vi "Log Error.vi"(8 "error in (no error)":errorcluster, 9 "error":errorcluster, 10 "state":T1, 11 "Dispatcher in":refnum<class "Dispatcher Thread.lvclass">) -> (0 "error out":errorcluster, 3 "Dispatcher out":refnum<class "Dispatcher Thread.lvclass">)   [LabVIEW 2017, in "DSF Core.lvlib" / "Dispatcher Thread.lvclass"]
uses:
  Dispatcher Thread.lvclass
  C:/Git/DSF/Core/Classes/Thread/Thread.lvclass
  Interface/Dispatcher/Command.ctl
  Thread.lvclass/Thread.ctl
  <vilib>/NI/Memory Manager/Classes/Pointer/Pointer.lvclass/Pointer.ctl
  Dispatcher Thread.lvclass/Dispatcher Thread.ctl
  Interface/Logging/Command Data.ctl
  Interface/Logging/Command.ctl
  Interface/Logging/Parameters.ctl
  Interface/Logging/Dispatcher State Parameters.ctl
  Interface/Interface.lvclass/Interface.ctl
  Interface/Send Command.vi
  Interface/Write RT FIFO.vi
  <vilib>/NI/Memory Manager/Classes/Pointer/Write.vi
  <vilib>/NI/Memory Manager/Classes/Pointer/Write 1D U8.vi
  <vilib>/NI/Memory Manager/Classes/Pointer/Clear.vi
  <vilib>/NI/Memory Manager/Classes/Pointer/Write (No Check).vi
  <vilib>/NI/Memory Manager/Classes/Pointer/Write (No Check) 1D U8.vi
  <vilib>/NI/Memory Manager/Classes/Pointer/Check Move.vi
  <vilib>/NI/Memory Manager/Classes/Pointer/Check Null Pointer.vi
  <vilib>/NI/Memory Manager/Classes/Pointer/Clear (No Check).vi
  <vilib>/NI/Memory Manager/Classes/Pointer/Check Length.vi
  <vilib>/NI/Memory Manager/Classes/Pointer/Check Count.vi
  <vilib>/NI/Memory Manager/Classes/Pointer/Check Bounds (Power of 2).vi
  <vilib>/NI/Memory Manager/Classes/Pointer/Errors.vi
  <vilib>/NI/Memory Manager/Classes/Pointer/Null Pointer.vi
  <vilib>/NI/Memory Manager/Classes/Pointer/Is Null.vi
  <vilib>/NI/Memory Manager/Classes/Pointer/Get Size.vi
  <vilib>/NI/Memory Manager/Classes/Pointer/Check Bounds (Pointer).vi
  <vilib>/NI/Memory Manager/Classes/Pointer/Out of Bounds.vi
  <vilib>/NI/Memory Manager/Classes/Pointer/Check Bounds.vi
  <vilib>/NI/Memory Manager/Classes/Pointer/Create Error.vi
  <vilib>/NI/Memory Manager/Classes/Pointer/Write Pointer Size to Error.vi
  <vilib>/NI/Memory Manager/Classes/Pointer/Check Bounds (Buffer).vi
  <vilib>/NI/Memory Manager/Constants/Constants.vi
  <vilib>/NI/Memory Manager/Constants/Library Name.vi
  <vilib>/NI/Memory Manager/Classes/Pointer/Pointer Error Info.vi
  <vilib>/NI/Memory Manager/Constants/Pointer Class Name.vi
  <vilib>/NI/Memory Manager/Classes/Pointer/Buffer Underflow.vi
  Pointers/Error/Error Pointer.lvclass
  C:/Program Files (x86)/National Instruments/LabVIEW 2017/vi.lib/NI/Memory Manager/Classes/Pointer/Pointer.lvclass
  Interface/Logging/Logging Interface.lvclass
  C:/Git/DSF/Core/Classes/Interface/Interface.lvclass
  Interface/Errors.vi
  Interface/Dispatcher/Command Timeout.vi
  VIs/VI Name.vi
  <vilib>/NI/Memory Manager/VIs/Write String to Source.vi
  <vilib>/NI/Memory Manager/VIs/Write Numeric to Source.vi
  <vilib>/NI/Memory Manager/VIs/Write Numeric Scalar to Source (Base10 U64).vi
  <vilib>/NI/Memory Manager/VIs/Set Error Source.vi
  <vilib>/NI/Memory Manager/VIs/Set Error Code.vi
  <vilib>/NI/Memory Manager/VIs/Set Error Status.vi
  <vilib>/NI/Memory Manager/VIs/New Error Cluster.vi
  <vilib>/NI/Memory Manager/VIs/New Error Cluster (512B).vi
  Interface/Logging/Send Logging Command.vi
  Interface/Dispatcher/Dispatcher Interface.lvclass
  Thread.lvclass
  <vilib>/NI/Memory Manager/Classes/Pointer/Pointer.lvclass
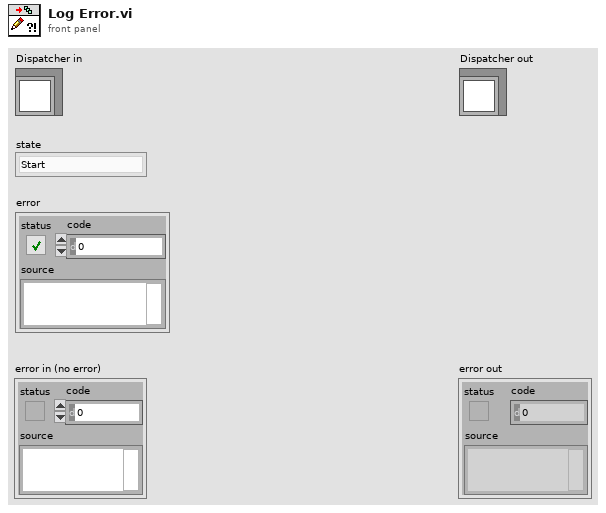
[diagram p1: front panel]
types:
  T1 = typedef "DSF Core.lvlib/Dispatcher Interface.lvclass/Command.ctl" = enum8{"Start", "Rx", "Tx", "Set Inline Buffer", "Shutdown"}
  T2 = typedef "DSF Core.lvlib/Logging Interface.lvclass/Parameters.ctl" = cluster{"arg1":u64, "arg2":u64}
  T3 = typedef "DSF Core.lvlib/Logging Interface.lvclass/Dispatcher State Parameters.ctl" = cluster{"state":T1, "unused":u8, "unused 2":u16, "unused 3":u32, "error pointer":u64}
  T4 = typedef "DSF Core.lvlib/Logging Interface.lvclass/Command.ctl" = enum8{"Start", "Log Framework State", "Log Plugin State", "Log Dispatcher State", "Log Framework Error", "Log Plugin Error", "Log Dispatcher Error", "Shutdown"}
  T5 = typedef "DSF Core.lvlib/Logging Interface.lvclass/Command Data.ctl" = cluster{"Command":T4, "Parameters":T2}
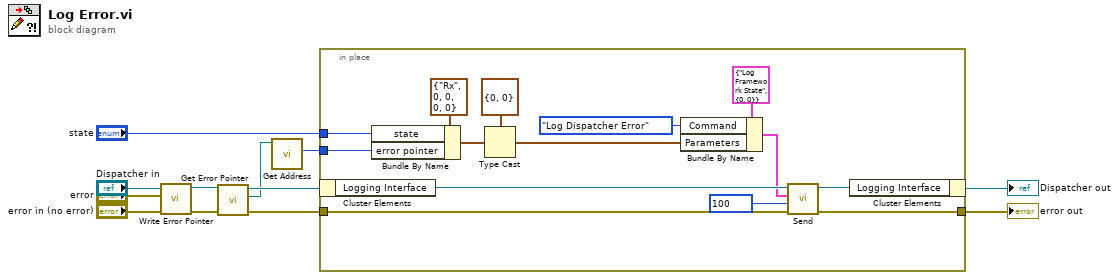
[diagram p0: block diagram]
diagram:
  n1 = call "Write Error Pointer.vi"("error in (no error)"="error in (no error)", "error"="error", "Thread in"="Dispatcher in") -> ("error out"=w3:errorcluster, "Thread out"=w2:refnum<class "Dispatcher Thread.lvclass">)  [unwired: 7 in]
  n2 = call "Get Error Pointer.vi"("Thread in"=w2) -> ("error pointer"=w8:refnum<class "Error Pointer.lvclass">, "Thread out"=w9:refnum<class "Dispatcher Thread.lvclass">)  [unwired: 9 in]
  n3 = call <vilib>:"Get Address.vi"("Pointer in"=w8) -> ("address"=w7:u64)  [unwired: 9 in, 1 out]
  n4 = in-place {
    in-place-border: [w21] -> w11
    in-place-border: w3 -> [w19]
    in-place-border: "state" -> [w14]
    in-place-border: w7 -> [w12]
    n5 = in-place-cluster #1(w9) -> ("Logging Interface"=w25:refnum<class "Logging Interface.lvclass">)
    n6 = Bundle By Name(cluster=T3 {"state"=enum."Rx", "unused"=0, "unused 2"=0, "unused 3"=0, "error pointer"=0} ("Parameters"), "state"=w14, "error pointer"=w12) -> (w17:T3)
    n7 = Type Cast(type=T2 {"arg1"=0, "arg2"=0} ("Parameters"), x=w17) -> (*(type *) &x=w15:T2)
    n8 = Bundle By Name(cluster=T5 {"Command"=enum."Log Framework State", "Parameters"={"arg1"=0, "arg2"=0}} ("command"), "Command"=Command."Log Dispatcher Error", "Parameters"=w15) -> (w22:T5)
    n9 = call-poly "Send.vi"("error in (no error)"=w19, "timeout in ms (0)"=100, "command"=w22, "Logging Interface in"=w25) -> ("error out"=w21:errorcluster, "Logging Interface out"=w20:refnum<class "Logging Interface.lvclass">)  [unwired: 6 in]
    n10 = in-place-cluster #1("Logging Interface"=w20) -> (→"Dispatcher out":refnum<class "Dispatcher Thread.lvclass">)
  }
  "error out" <- w11
